vi "Read Sub Panel Productos.vi"(8 "error in (no error)":errorcluster, 11 "Productos in":refnum<class "Productos.lvclass">) -> (0 "error out":errorcluster, 2 "Sub Panel Productos":refnum<vi>, 3 "Productos out":refnum<class "Productos.lvclass">)   [LabVIEW 2020, in "Productos.lvlib" / "Productos.lvclass"]
uses:
  Productos.lvclass
  Productos.lvclass/Productos.ctl
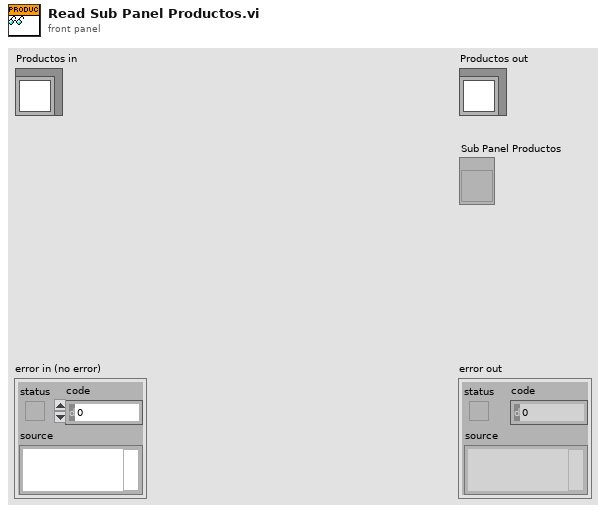
[diagram p1: front panel]
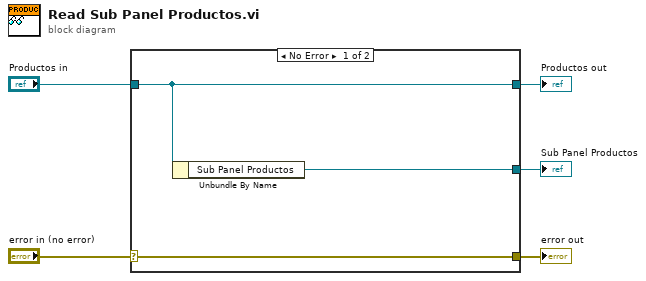
[diagram p0: block diagram]
diagram:
  n1 = case shown="No Error" "error in (no error)" {
    selector: "error in (no error)" -> [w8 w9]
    tunnel: [w8 w9] -> w4
    tunnel: [w7 w10] -> w2
    tunnel: "Productos in" -> [w7 w10]
    tunnel: [w6 _] -> w1
    frame No Error {
      n2 = Unbundle By Name(w7) -> ("Sub Panel Productos"=w6:refnum<vi>)
    }
    frame Error {
    }
  }
  "error out" <- w4
  "Productos out" <- w2
  "Sub Panel Productos" <- w1
